vi "Read Stop Event.vi"(11 "IEventHandler in":refnum<class "IEventHandler.lvclass">) -> (2 "Stop! Event":refnum<user-event>)   [LabVIEW 2018, in "MVA Framework.lvlib" / "ActorEvents.lvlib" / "IEventHandler.lvclass"]
doc: "读取停止事件"
uses:
  IEventHandler.lvclass
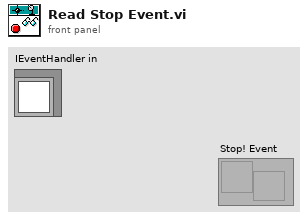
[diagram p1: front panel]
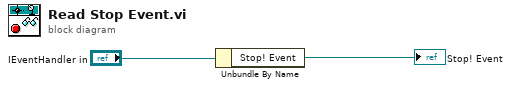
[diagram p0: block diagram]
diagram:
  n1 = Unbundle By Name("IEventHandler in") -> ("Stop! Event"=→"Stop! Event":refnum<user-event>)
